vi "Pre Launch Init.vi"(11 "TDMS Data Logger Actor in":refnum<class "TDMS Data Logger Actor.lvclass">) -> (0 "error out":errorcluster, 3 "TDMS Data Logger Actor out":refnum<class "TDMS Data Logger Actor.lvclass">)   [LabVIEW 2024, in "TDMS Data Logger Actor.lvlib" / "TDMS Data Logger Actor.lvclass"]
doc: "<p>(<strong>Filename</strong>: <span class=\"dnl\">Actor Framework.lvlib:Actor.lvclass:Pre Launch Init.vi</span>)</p>\n<p>Defines behavior that occurs after the <a href=\"nihelplauncher://docs/csh?context=lvcore_lvcomm_af_launch_nested_actor\">Launch Nested Actor</a> method is invoked but before the actor's Actor Core method begins running.</p>\n<p>By default, this method does nothing. A descendant class may override it to define behavior.</p>"
uses:
  TDMS Data Logger Actor.lvclass
  TDMS Data Logger Actor.lvclass/TDMS Data Logger Actor.ctl
  <vilib>/ActorFramework/Actor/Actor.lvclass
  Logging Data Interface/Logging Data Interface/Logging Data Interface.lvclass
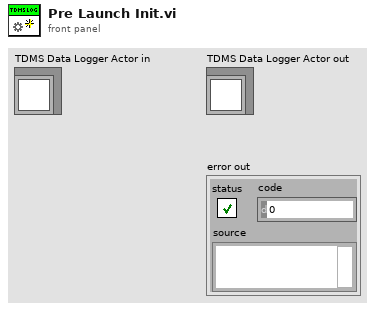
[diagram p1: front panel]
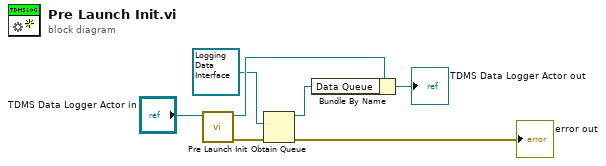
[diagram p0: block diagram]
diagram:
  n1 = call-parent "Pre Launch Init.vi"("Actor in"="TDMS Data Logger Actor in") -> ("error out"=w6:errorcluster, "Actor out"=w4:refnum<class "TDMS Data Logger Actor.lvclass">)  [unwired: 9 in]
  n2 = Obtain Queue(element data type=refnum<class "Logging Data Interface.lvclass"> refnum ("Logging Data Interface.lvlib:Logging Data Interface.lvclass"), error in (no error)=w6) -> (queue out=w1:refnum<queue>, error out=→"error out":errorcluster)  [unwired: 3 in, 1 out]
  n3 = Bundle By Name(cluster=w4, "Data Queue"=w1) -> (→"TDMS Data Logger Actor out":refnum<class "TDMS Data Logger Actor.lvclass">)
